vi "DAC Stop.vi"(8 "error in (no error)":errorcluster, 11 "DAC Keller PAA25 in":refnum<class "DAC Keller PAA25.lvclass">) -> (0 "error out":errorcluster, 3 "DAC Keller PAA25 out":refnum<class "DAC Keller PAA25.lvclass">)   [LabVIEW 2019, in "DAC.lvlib" / "DAC Keller PAA25.lvclass"]
uses:
  DAC Keller PAA25.lvclass
  C:/Users/wg/Documents/LV_Projects/test-stand/App/DAC/DAC.lvclass
  DAC.lvclass/DAC.ctl
  DAC Keller PAA25.lvclass/DAC Keller PAA25.ctl
  DAC.lvclass
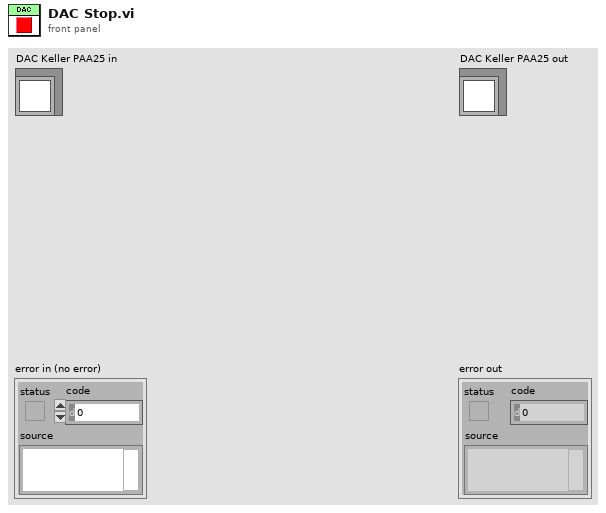
[diagram p1: front panel]
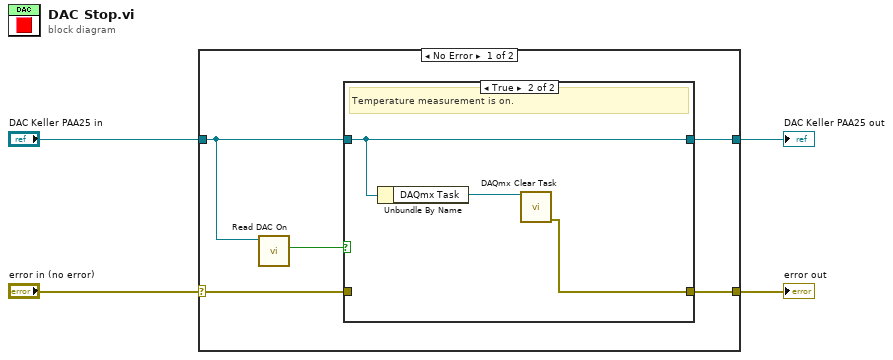
[diagram p0: block diagram]
diagram:
  n1 = case shown="No Error" "error in (no error)" {
    selector: "error in (no error)" -> [w6 w16]
    tunnel: [w5 w16] -> w1
    tunnel: [w7 w15] -> w3
    tunnel: "DAC Keller PAA25 in" -> [w9 w15]
    frame No Error {
      n2 = call "Read DAC On.vi"("DAC in"=w9) -> ("DAC On"=w8:bool)  [unwired: 8 in, 2 out]
      n3 = case shown="True" w8 {
        tunnel: w9 -> [w11 w14]
        tunnel: [w11 w14] -> w7
        tunnel: w6 -> [w10 _]
        tunnel: [w10 w12] -> w5
        frame False {
          # "Temperature measurement is off."
        }
        frame True {
          # "Temperature measurement is on."
          n4 = Unbundle By Name(w14) -> ("DAQmx Task"=w13:refnum<k21>)
          n5 = call <vilib>:"DAQmx Clear Task.vi"("task in"=w13) -> ("error out"=w12:errorcluster)  [unwired: 14 in]
        }
      }
    }
    frame Error {
    }
  }
  "error out" <- w1
  "DAC Keller PAA25 out" <- w3
